vi "Update GlobalStop.WriterState.vi"(8 "error in":errorcluster, 11 "RunState":bool) -> (0 "error out":errorcluster)   [LabVIEW 2021, in "XNET-CAN-Signal-Logger.lvlib"]
uses:
  XNET-CAN-Signal-Logger.lvlib
  Global Variables.vi
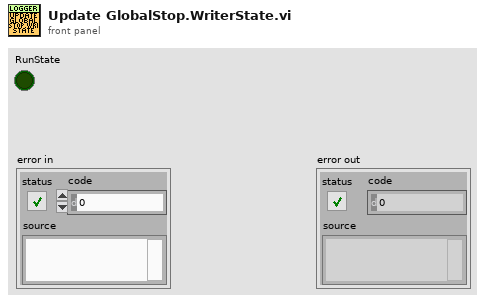
[diagram p1: front panel]
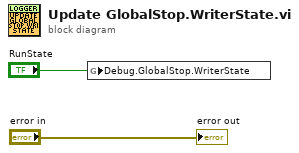
[diagram p0: block diagram]
diagram:
  n1 = global write "Global Variables.vi" "Debug.GlobalStop.WriterState"("RunState") -> ()
  "error out" <- "error in"
